vi "text bool to t f dont care.vi"(8 "error in (no error)":errorcluster, 9 "bits":bool[][](array[boolean]), 10 "acceptable results":string[](array[string])) -> (0 "error out":errorcluster, 2 "acceptable result":bool)   [LabVIEW 2020]
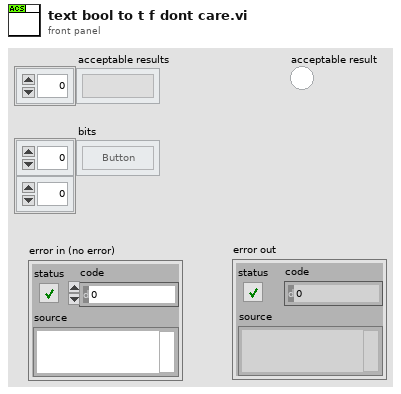
[diagram p1: front panel]
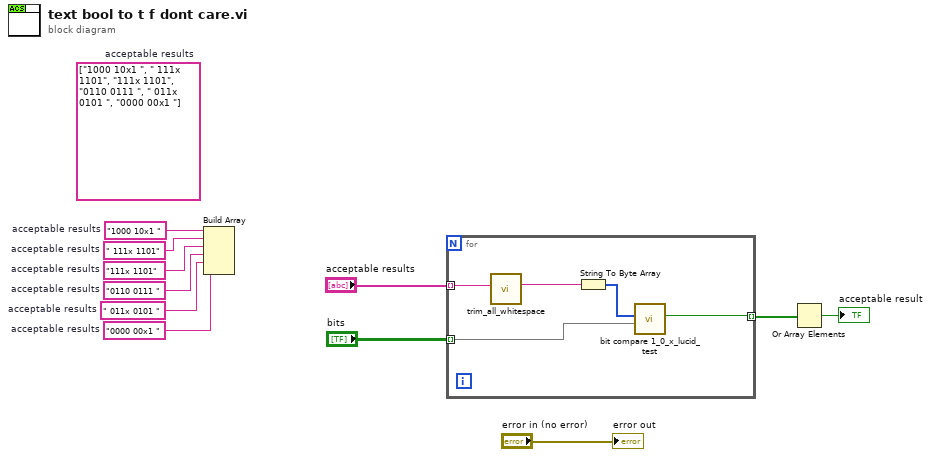
[diagram p0: block diagram]
diagram:
  (unwired) string[] ["1000 10x1 ", " 111x 1101", "111x 1101", "0110 0111 ", " 011x 0101 ", "0000 00x1 "]  # acceptable results
  w6 = "0000 00x1 "  # acceptable results
  w7 = " 011x 0101 "  # acceptable results
  w8 = "0110 0111 "  # acceptable results
  w9 = "111x 1101"  # acceptable results
  w10 = " 111x 1101"  # acceptable results
  w11 = "1000 10x1 "  # acceptable results
  n1 = Build Array(w11, w10, w9, w8, w7, w6) -> ()  [unwired: 1 out]
  n2 = for {
    tunnel: "acceptable results" -> [w14] mode=indexing
    tunnel: "bits" -> [w13] mode=indexing
    tunnel: [w12] -> w5 mode=indexing
    n3 = call "trim_all_whitespace.vi"("String"=w14) -> ("Trimmed String"=w15:string)  [unwired: 10 in]
    n4 = String To Byte Array(string=w15) -> (unsigned byte array=w16:u8[])
    n5 = call "bit compare 1_0_x_lucid_test.vi"("Input"=w13, "unsigned byte array"=w16) -> ("x = y?"=w12:bool)  [unwired: 9 in]
  }
  n6 = Or Array Elements(Boolean array=w5) -> (logical OR=→"acceptable result":bool)
  "error out" <- "error in (no error)"
